vi "AUTON_Index.vi"(0 "Auton Array":dbl[][](array[numeric]), 5 "MeasuredHeading":dbl, 7 "LeftEncoder":dbl, 9 "RightEncoder":dbl) -> (4 "Left Drive":dbl, 6 "Right Drive":dbl, 8 "Indexer":dbl, 10 "Shooter Elevation":dbl, 13 "Flipper":dbl, 14 "Roller":dbl, 15 "Shooter Wheels":dbl)   [LabVIEW 2012]
uses:
  Robot Global Data.vi
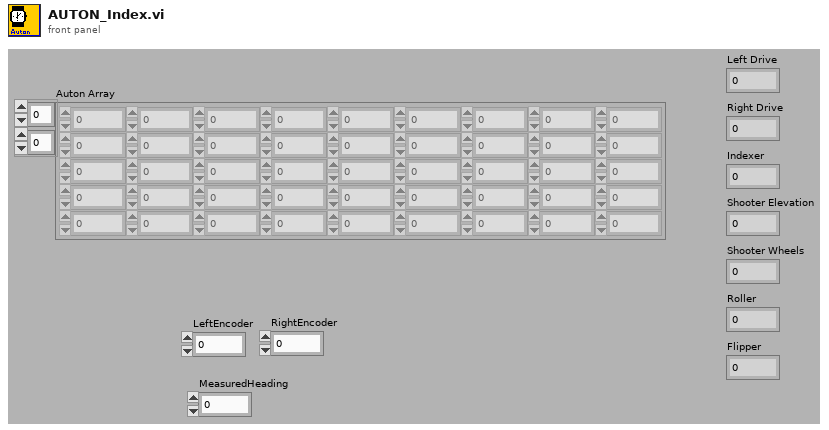
[diagram p1: front panel]
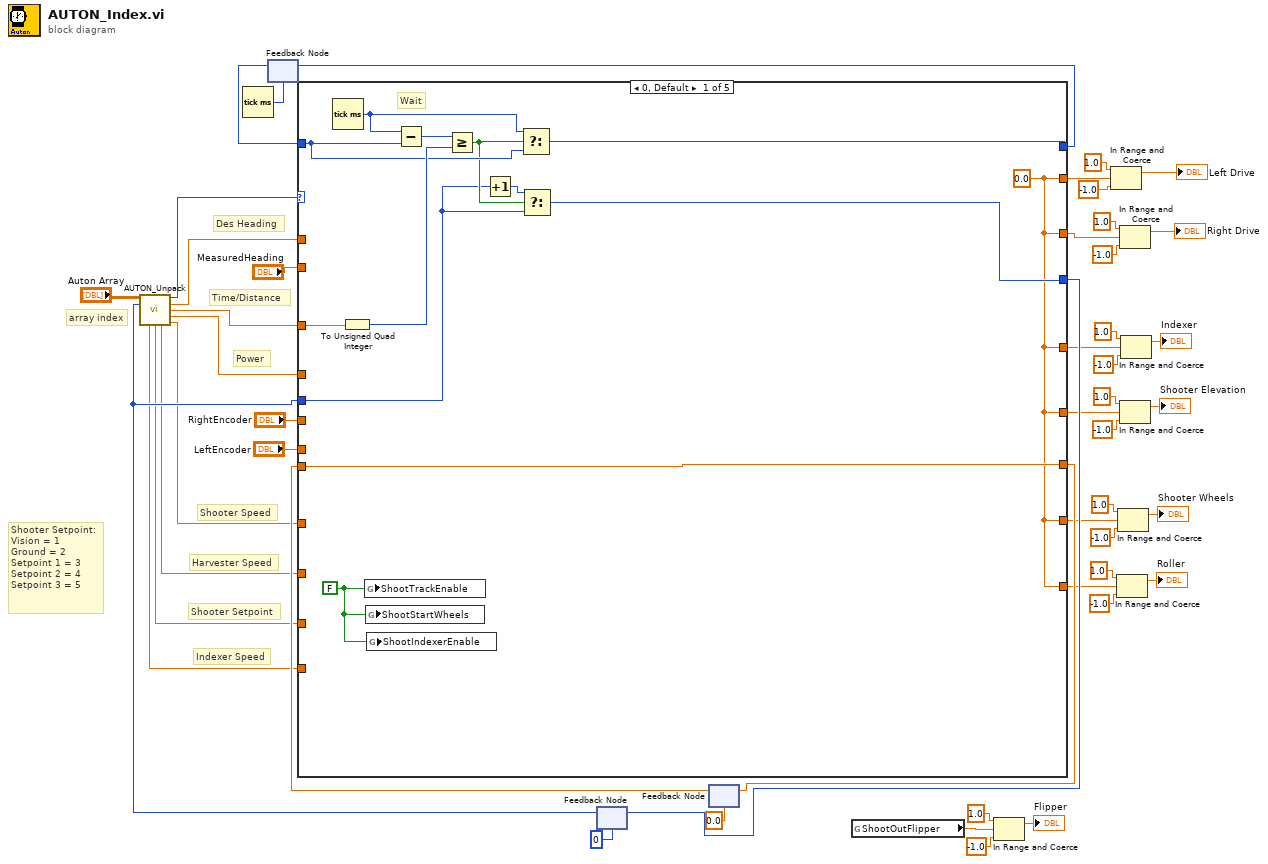
[diagram p0: block diagram]
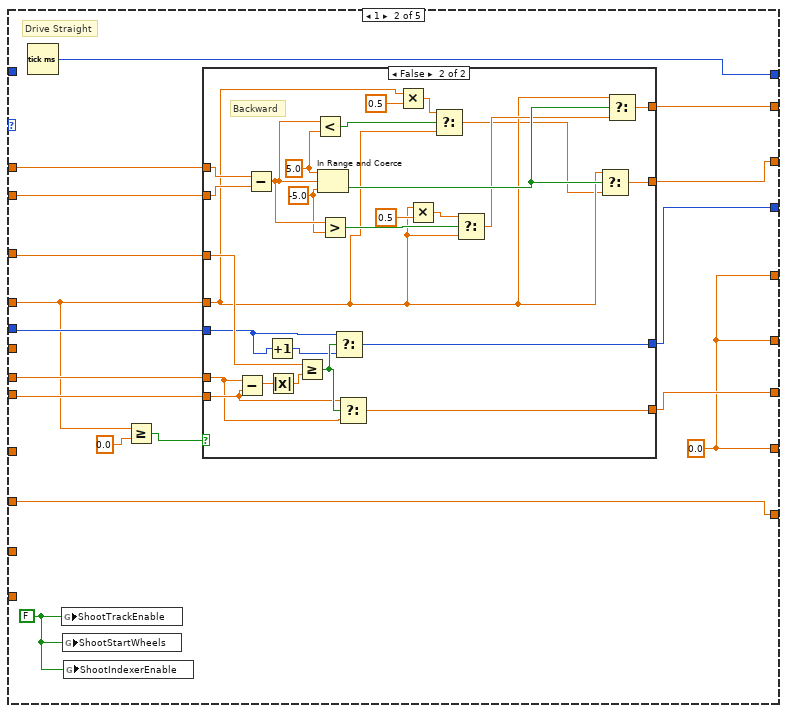
[diagram p2: hidden frame]
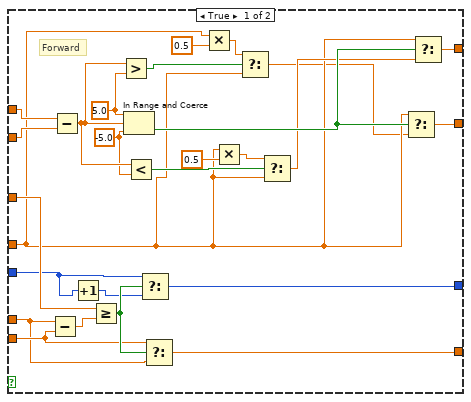
[diagram p3: hidden frame]
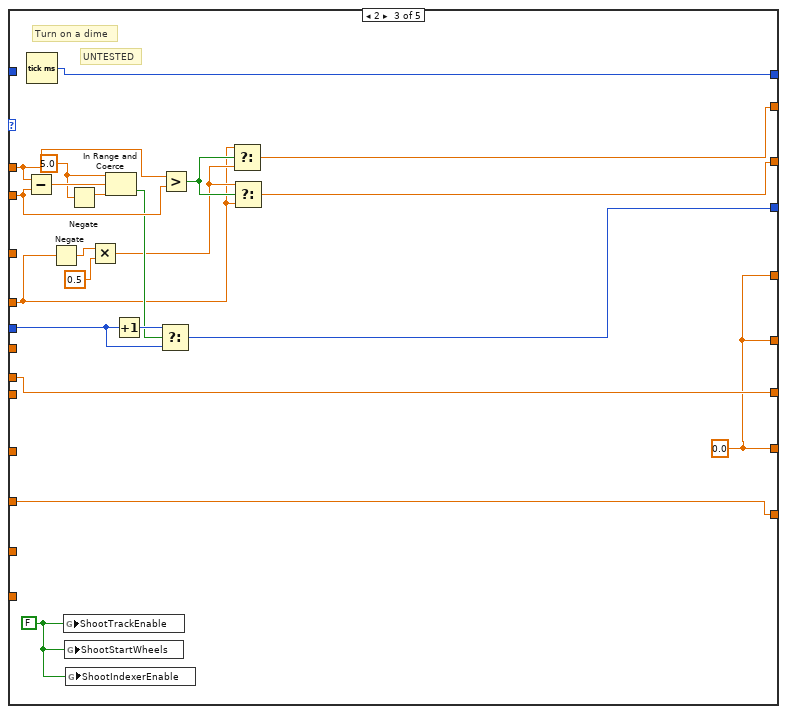
[diagram p4: hidden frame]
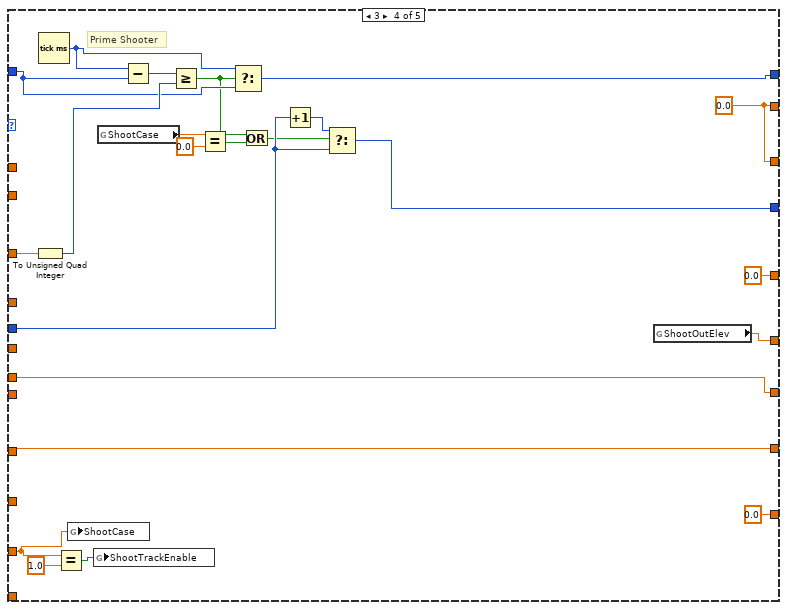
[diagram p5: hidden frame]
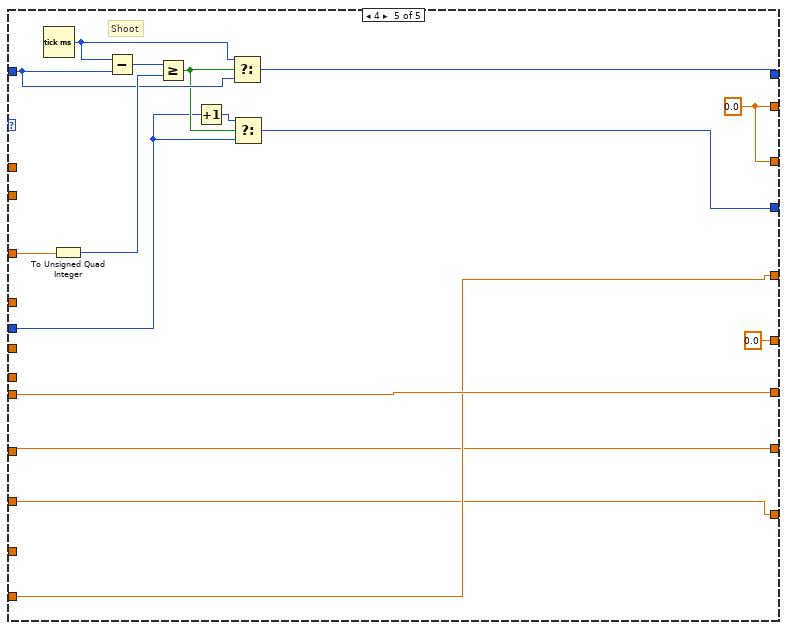
[diagram p6: hidden frame]
diagram:
  # "Shooter Setpoint:\nVision = 1\nGround = 2\nSetpoint 1 = 3\nSetpoint 2 = 4\nSetpoint 3 = 5"
  # "Indexer Speed"
  # "Shooter Speed"
  # "Shooter Setpoint"
  # "Harvester Speed"
  # "Des Heading"
  # "Time/Distance"
  # "Power"
  # "array index"
  n1 = Tick Count (ms)() -> (millisecond timer value=w46:u32)
  n2 = feedback #1(w46) -> (w48:u32)
  n3 = feedback #2(0) -> (w25:i32)
  n4 = call "AUTON_Unpack.vi"("all rows"="Auton Array", "Index"=w25) -> ("Primitive ID"=w29:i16, "Desired Heading"=w27:dbl, "Time/Distance"=w26:dbl, "Power"=w28:dbl, "Indexer Speed"=w21:dbl, "Shooter Setpoint"=w22:dbl, "Harvester Speed"=w23:dbl, "Shooter Speed"=w24:dbl)  [unwired: 6 in]
  n5 = feedback #3(0.0) -> (w31:dbl)
  n6 = case shown="0, Default" w29 {
    tunnel: [w54 w77 w148 w168 w184] -> w34
    tunnel: w25 -> [w55 w72 w151 w159 w185]
    tunnel: [w62 w69 w153 w157 w192] -> w36
    tunnel: w48 -> [w59 _ _ w158 w189]
    tunnel: w26 -> [w53 w78 _ w160 w183]
    tunnel: w27 -> [_ w76 w143 _ _]
    tunnel: [w51 w74 w149 w176 w181] -> w44
    tunnel: [w51 w73 w150 w176 w181] -> w37
    tunnel: w28 -> [_ w68 w136 _ _]
    tunnel: "LeftEncoder" -> [_ w70 w147 w175 _]
    tunnel: "MeasuredHeading" -> [_ w75 w142 _ _]
    tunnel: "RightEncoder" -> [_ _ _ _ _]
    tunnel: w31 -> [w52 w71 _ _ w182]
    tunnel: [w52 w79 w147 w175 w182] -> w30
    tunnel: w24 -> [_ _ _ w174 w178]
    tunnel: w23 -> [_ w63 w133 _ w177]
    tunnel: w22 -> [_ _ _ w164 _]
    tunnel: w21 -> [_ _ _ _ w180]
    tunnel: [w51 w63 w133 0.0 ("Harvester Speed") w177] -> w5
    tunnel: [w51 w65 w134 w174 w178] -> w4
    tunnel: [w51 w65 w134 w171 0.0 ("ShootOutElev")] -> w3
    tunnel: [w51 w65 w134 0.0 ("Numeric") w180] -> w2
    frame 0, Default {
      w50 = FALSE ("ShootTrackEnable")
      w51 = 0.0 ("Numeric")
      # "Wait"
      n7 = Tick Count (ms)() -> (millisecond timer value=w58:u32)
      n8 = To Unsigned Quad Integer(1:w53) -> (0:w60:u64)
      n9 = global write "Robot Global Data.vi" "ShootTrackEnable"(w50) -> ()
      n10 = global write "Robot Global Data.vi" "ShootStartWheels"(w50) -> ()
      n11 = global write "Robot Global Data.vi" "ShootIndexerEnable"(w50) -> ()
      n12 = Subtract(x=w58, y=w59) -> (x-y=w61:u32)
      n13 = Greater Or Equal?(x=w61, y=w60) -> (x >= y?=w57:bool)
      n14 = Increment(x=w55) -> (x+1=w56:i32)
      n15 = Select(t=w58, s=w57, f=w59) -> (s? t:f=w62:u32)
      n16 = Select(t=w56, s=w57, f=w55) -> (s? t:f=w54:i32)
    }
    frame 1 {
      w64 = FALSE ("ShootTrackEnable")
      w65 = 0.0 ("Numeric")
      # "Drive Straight"
      n17 = Tick Count (ms)() -> (millisecond timer value=w69:u32)
      n18 = global write "Robot Global Data.vi" "ShootTrackEnable"(w64) -> ()
      n19 = global write "Robot Global Data.vi" "ShootStartWheels"(w64) -> ()
      n20 = global write "Robot Global Data.vi" "ShootIndexerEnable"(w64) -> ()
      n21 = Greater Or Equal?(x=w68, y=0.0) -> (x >= y?=w66:bool)
      n22 = case shown="False" w66 {
        tunnel: [w105 w132] -> w79
        tunnel: w78 -> [w103 w131]
        tunnel: [w101 w129] -> w77
        tunnel: w76 -> [w100 w128]
        tunnel: w75 -> [w99 w127]
        tunnel: [w97 w125] -> w74
        tunnel: [w96 w124] -> w73
        tunnel: w68 -> [w85 w113]
        tunnel: w72 -> [w82 w110]
        tunnel: w71 -> [w81 w109]
        tunnel: w70 -> [w80 w108]
        frame True {
          w93 = -5.0 ("lower limit")
          w95 = 5.0 ("upper limit")
          # "Forward"
          n23 = Subtract(x=w80, y=w81) -> (x-y=w104:dbl)
          n24 = Subtract(x=w100, y=w99) -> (x-y=w94:dbl)
          n25 = Increment(x=w82) -> (x+1=w83:i32)
          n26 = Greater Or Equal?(x=w103, y=w104) -> (x >= y?=w102:bool)
          n27 = Greater?(x=w94, y=w95) -> (0:w88:bool)
          n28 = In Range and Coerce(upper limit=w95, x=w94, lower limit=w93) -> (In Range?=w98:bool)  [unwired: 1 out]
          n29 = Less?(x=w94, y=w93) -> (x < y?=w92:bool)
          n30 = Select(t=w82, s=w102, f=w83) -> (s? t:f=w101:i32)
          n31 = Select(t=w81, s=w102, f=w80) -> (s? t:f=w105:dbl)
          n32 = Multiply(x=w85, y=0.5) -> (x*y=w87:dbl)
          n33 = Multiply(x=w85, y=0.5) -> (x*y=w90:dbl)
          n34 = Select(t=w87, s=w88, f=w85) -> (s? t:f=w84:dbl)
          n35 = Select(t=w90, s=w92, f=w85) -> (s? t:f=w89:dbl)
          n36 = Select(t=w85, s=w98, f=w84) -> (s? t:f=w96:dbl)
          n37 = Select(t=w85, s=w98, f=w89) -> (s? t:f=w97:dbl)
        }
        frame False {
          w121 = -5.0 ("lower limit")
          w123 = 5.0 ("upper limit")
          # "Backward"
          n38 = Subtract(x=w108, y=w109) -> (x-y=w106:dbl)
          n39 = Subtract(x=w128, y=w127) -> (x-y=w122:dbl)
          n40 = Increment(x=w110) -> (x+1=w111:i32)
          n41 = Absolute Value(x=w106) -> (abs(x)=w107:dbl)
          n42 = Greater Or Equal?(x=w131, y=w107) -> (x >= y?=w130:bool)
          n43 = Less?(x=w122, y=w123) -> (x < y?=w116:bool)
          n44 = In Range and Coerce(upper limit=w123, x=w122, lower limit=w121) -> (In Range?=w126:bool)  [unwired: 1 out]
          n45 = Greater?(x=w122, y=w121) -> (0:w120:bool)
          n46 = Select(t=w110, s=w130, f=w111) -> (s? t:f=w129:i32)
          n47 = Select(t=w109, s=w130, f=w108) -> (s? t:f=w132:dbl)
          n48 = Multiply(x=w113, y=0.5) -> (x*y=w115:dbl)
          n49 = Multiply(x=w113, y=0.5) -> (x*y=w118:dbl)
          n50 = Select(t=w115, s=w116, f=w113) -> (s? t:f=w112:dbl)
          n51 = Select(t=w118, s=w120, f=w113) -> (s? t:f=w117:dbl)
          n52 = Select(t=w113, s=w126, f=w112) -> (s? t:f=w124:dbl)
          n53 = Select(t=w113, s=w126, f=w117) -> (s? t:f=w125:dbl)
        }
      }
    }
    frame 2 {
      w134 = 0.0 ("Numeric")
      w135 = FALSE ("ShootTrackEnable")
      w144 = 5.0 ("upper limit")
      # "UNTESTED"
      # "Turn on a dime"
      n54 = Subtract(x=w143, y=w142) -> (x-y=w146:dbl)
      n55 = Tick Count (ms)() -> (millisecond timer value=w153:u32)
      n56 = Negate(x=w136) -> (-x=w139:dbl)
      n57 = global write "Robot Global Data.vi" "ShootTrackEnable"(w135) -> ()
      n58 = global write "Robot Global Data.vi" "ShootStartWheels"(w135) -> ()
      n59 = global write "Robot Global Data.vi" "ShootIndexerEnable"(w135) -> ()
      n60 = Negate(x=w144) -> (-x=w145:dbl)
      n61 = Multiply(x=w139, y=0.5) -> (x*y=w137:dbl)
      n62 = In Range and Coerce(upper limit=w144, x=w146, lower limit=w145) -> (In Range?=w141:bool)  [unwired: 1 out]
      n63 = Increment(x=w151) -> (x+1=w152:i32)
      n64 = Select(t=w152, s=w141, f=w151) -> (s? t:f=w148:i32)
      n65 = Greater?(x=w143, y=w142) -> (0:w140:bool)
      n66 = Select(t=w136, s=w140, f=w137) -> (s? t:f=w149:dbl)
      n67 = Select(t=w137, s=w140, f=w136) -> (s? t:f=w150:dbl)
    }
    frame 3 {
      w176 = 0.0 ("Power")
      # "Prime Shooter"
      n68 = To Unsigned Quad Integer(1:w160) -> (0:w162:u64)
      n69 = Tick Count (ms)() -> (millisecond timer value=w161:u32)
      n70 = Equal?(x=w164, y=1.0) -> (x = y?=w165:bool)
      n71 = global write "Robot Global Data.vi" "ShootCase"(w164) -> ()
      n72 = global write "Robot Global Data.vi" "ShootTrackEnable"(w165) -> ()
      n73 = global read "Robot Global Data.vi" "ShootCase"() -> (w170:dbl)
      n74 = Subtract(x=w161, y=w158) -> (x-y=w163:u32)
      n75 = Greater Or Equal?(x=w163, y=w162) -> (x >= y?=w154:bool)
      n76 = Equal?(x=w170, y=0.0) -> (x = y?=w156:bool)
      n77 = Select(t=w161, s=w154, f=w158) -> (s? t:f=w157:u32)
      n78 = Or(x=w154, y=w156) -> (x .or. y?=w155:bool)
      n79 = Increment(x=w159) -> (x+1=w167:i32)
      n80 = Select(t=w167, s=w155, f=w159) -> (s? t:f=w168:i32)
      n81 = global read "Robot Global Data.vi" "ShootOutElev"() -> (w171:dbl)
    }
    frame 4 {
      w181 = 0.0 ("Numeric")
      # "Shoot"
      n82 = Tick Count (ms)() -> (millisecond timer value=w188:u32)
      n83 = To Unsigned Quad Integer(1:w183) -> (0:w190:u64)
      n84 = Subtract(x=w188, y=w189) -> (x-y=w191:u32)
      n85 = Greater Or Equal?(x=w191, y=w190) -> (x >= y?=w187:bool)
      n86 = Increment(x=w185) -> (x+1=w186:i32)
      n87 = Select(t=w188, s=w187, f=w189) -> (s? t:f=w192:u32)
      n88 = Select(t=w186, s=w187, f=w185) -> (s? t:f=w184:i32)
    }
  }
  n89 = feedback-in #1(w36) -> ()
  n90 = feedback-in #2(w34) -> ()
  n91 = feedback-in #3(w30) -> ()
  n92 = global read "Robot Global Data.vi" "ShootOutFlipper"() -> (w1:dbl)
  n93 = In Range and Coerce(upper limit=1.0, x=w1, lower limit=-1.0) -> (coerced(x)=→"Flipper":dbl)  [unwired: 1 out]
  n94 = In Range and Coerce(upper limit=1.0, x=w44, lower limit=-1.0) -> (coerced(x)=→"Left Drive":dbl)  [unwired: 1 out]
  n95 = In Range and Coerce(upper limit=1.0, x=w5, lower limit=-1.0) -> (coerced(x)=→"Roller":dbl)  [unwired: 1 out]
  n96 = In Range and Coerce(upper limit=1.0, x=w4, lower limit=-1.0) -> (coerced(x)=→"Shooter Wheels":dbl)  [unwired: 1 out]
  n97 = In Range and Coerce(upper limit=1.0, x=w37, lower limit=-1.0) -> (coerced(x)=→"Right Drive":dbl)  [unwired: 1 out]
  n98 = In Range and Coerce(upper limit=1.0, x=w3, lower limit=-1.0) -> (coerced(x)=→"Shooter Elevation":dbl)  [unwired: 1 out]
  n99 = In Range and Coerce(upper limit=1.0, x=w2, lower limit=-1.0) -> (coerced(x)=→"Indexer":dbl)  [unwired: 1 out]
